vi "UHR-Fleezers Control (host) -TL - oscillation.vi"(0 "Tab Control":T5(tab)) -> ()   [LabVIEW 2013] (continued)
            n248 = VISA Write(VISA resource name=w463, write buffer=w464) -> ()  [unwired: 1 in, 3 out]
          }
          frame #4 {
            n249 = Wait (ms)(milliseconds to wait=u32 200) -> ()  [unwired: 1 out]
          }
          frame #5 {
            # "Change the trajectory mode to Jog"
            n250 = local read "ESP Port"() -> (w468:refnum<visa-resource-name>)
            n251 = Concatenate Strings("1TJ3;\n2TJ3;\n3TJ3" ("Substring"), "\r") -> (w471:string)
            n252 = VISA Write(VISA resource name=w468, write buffer=w471) -> ()  [unwired: 1 in, 3 out]
          }
        }
      }
      event "Capture": Value Change {
        n253 = event-data() -> ()  [unwired: 1 in, 5 out]
        n254 = local read "Capture Locations"() -> (w472:i32)
        n255 = local read "Z Pos Pos"() -> (w473:string)
        n256 = local read "X Pos"() -> (w475:string)
        n257 = local read "Y Pos"() -> (w474:string)
        n258 = case shown="1" w472 {
          selector: w472 -> [w479 w486 w493 w500]
          tunnel: w475 -> [w482 w489 w496 w503]
          tunnel: w474 -> [w481 w488 w495 w502]
          tunnel: w473 -> [w480 w487 w494 w501]
          frame 0, Default {
            # "Capture Top Dispensor Location"
            n259 = local read "Location Matrix"() -> (w478:string[][])
            n260 = Build Array(w482, w481, w480) -> (w477:string[])
            n261 = Replace Array Subset(array=w478, new element=w477, index (row)=w479) -> (w476:string[][])  [unwired: 1 in]
            n262 = local write "Location Matrix"(w476) -> ()
          }
          frame 1 {
            # "Capture Bottom Dispensor Location"
            n263 = local read "Location Matrix"() -> (w485:string[][])
            n264 = Build Array(w489, w488, w487) -> (w484:string[])
            n265 = Replace Array Subset(array=w485, new element=w484, index (row)=w486) -> (w483:string[][])  [unwired: 1 in]
            n266 = local write "Location Matrix"(w483) -> ()
          }
          frame 2 {
            # "Capture Experimental Region Location"
            n267 = local read "Location Matrix"() -> (w492:string[][])
            n268 = Build Array(w496, w495, w494) -> (w491:string[])
            n269 = Replace Array Subset(array=w492, new element=w491, index (row)=w493) -> (w490:string[][])  [unwired: 1 in]
            n270 = local write "Location Matrix"(w490) -> ()
          }
          frame 3 {
            # "Capture Other Location"
            n271 = local read "Location Matrix"() -> (w499:string[][])
            n272 = Build Array(w503, w502, w501) -> (w498:string[])
            n273 = Replace Array Subset(array=w499, new element=w498, index (row)=w500) -> (w497:string[][])  [unwired: 1 in]
            n274 = local write "Location Matrix"(w497) -> ()
          }
        }
      }
      event "Save": Value Change {
        # "reshape Location Matrix to 1-D array to write"
        n275 = event-data() -> ()  [unwired: 1 in, 5 out]
        n276 = local read "Location Matrix"() -> (w507:string[][])
        n277 = local read "Location path"() -> (w504:path)
        n278 = Reshape Array(w507, 12) -> (w505:string[])
        n279 = Write to Text File(file (use dialog)=w504, text=w505) -> ()  [unwired: 2 in, 3 out]
      }
      event "Activate Joystick": Value Change {
        # "Change the trajectory mode to Jog"
        n280 = event-data() -> ()  [unwired: 1 in, 5 out]
        n281 = disable-structure shown="Disabled" {
          frame Disabled {
            n282 = case shown="True" "Activate Joystick" {
              frame False {
              }
              frame True {
                # "Change the trajectory mode to Jog"
                n283 = local read "ESP Port"() -> (w516:refnum<visa-resource-name>)
                n284 = Concatenate Strings("1TJ3;\n2TJ3;\n3TJ3" ("Substring"), "\r") -> (w513:string)
                n285 = VISA Write(VISA resource name=w516, write buffer=w513) -> ()  [unwired: 1 in, 3 out]
              }
            }
          }
          frame Enabled {
          }
        }
        n286 = local read "ESP Port"() -> (w508:refnum<visa-resource-name>)
        n287 = Concatenate Strings("1TJ3;\n2TJ3;\n3TJ3" ("Substring"), "\r") -> (w511:string)
        n288 = VISA Write(VISA resource name=w508, write buffer=w511) -> ()  [unwired: 1 in, 3 out]
      }
    }
  }
  n289 = disable-structure shown="Disabled" {
    disable-tunnel: w2 -> [w545 _]
    frame Disabled {
      w540 = T17 0 items=["Grayscale (U8)", "Grayscale (I16)", "Grayscale (SGL)", "Complex (CSG)", "RGB (U32)", "HSL (U32)", "RGB (U64)", "Grayscale (U16)"] ("Image Type")
      n290 = call <vilib>:"IMAQ Init.vi"("Interface Name"="img0") -> ("error out"=w542:errorcluster, "IMAQ Session Out"=w544:refnum<k11>)  [unwired: 9 in]
      n291 = call <vilib>:"IMAQ Grab Setup.vi"("error in (no error)"=w542, "IMAQ Session In"=w544) -> ("error out"=w538:errorcluster, "IMAQ Session Out"=w539:refnum<k11>)  [unwired: 8 in]
      n292 = call "IMAQ Create"("Image Name"="untitled", "Image Type"=w540) -> ("New Image"=w537:T3)  [unwired: 3 in, 1 out]
      n293 = call <vilib>:"Application Directory.vi"() -> ("Application Directory"=w524:path)
      n294 = Build Path(base path=w524, name or relative path="_trap_screen_positions") -> (appended path=w532:path)
      n295 = Open/Create/Replace File(file path (use dialog)=w532, operation (0:open)=T23."open or create", access (0:read/write)=enum16{"read/write", "read-only", "write-only"}."read/write") -> (refnum out=w534:refnum<file>)  [unwired: 3 in, 2 out]
      n296 = local read "Trap Sets"() -> (w526:u32)
      n297 = for "Load trap positions on video screen from file." {
        N: w526 -> [_]
        tunnel: [w552] -> w527
        tunnel: w534 -> [w551]
        tunnel: [w548] -> w523 mode=indexing
        w550 = 4
        n298 = for {
          N: w550 -> [_]
          tunnel: [w556] -> w552
          tunnel: w551 -> [w555]
          tunnel: w550 -> [w554]
          tunnel: [w553] -> w549 mode=indexing
          n299 = Read from Binary File(5:w554, 11:w555) -> (2:w553:i32, 3:w556:refnum<file>)  [unwired: 4 in, 2 out]
        }
        n300 = Array To Cluster(array=w549) -> (cluster=w548:T27)
      }
      n301 = node-c288() -> (w547:T24)  [unwired: 4 in]
      n302 = timed-loop "acquire video and stage position" {
        timing: w547 -> [_]
        timing-out: [_] -> w546
        tunnel: w539 -> [w575]
        tunnel: w538 -> [w574]
        tunnel: w537 -> [w573]
        tunnel: [w572] -> w519
        tunnel: [w569] -> w520
        tunnel: [w570] -> w518
        tunnel: w545 -> [_]
        shift-right: [w566] -> w536
        shift-left: w523 -> [w567]
        tunnel: w526 -> [w564]
        stop <- w571 stop-if-true
        n303 = node-c288() -> ()  [unwired: 1 in, 1 out]
        n304 = event shown="[0] Timeout" {
          selector: _ -> [_ _ _ _]
          dyn-events: _ -> [_ _ _ _]
          timeout: 10 -> [_ _ _ _]
          tunnel: w575 -> [w586 w601 w610 w629]
          tunnel: w574 -> [w585 w603 w608 w631]
          tunnel: w573 -> [w584 w602 w609 w630]
          tunnel: [w583 w601 w610 w629] -> w572
          tunnel: [w576 w605 FALSE FALSE] -> w571
          tunnel: [w580 w603 w608 w631] -> w570
          tunnel: [w579 w602 w609 w630] -> w569
          tunnel: "radius" -> [_ _ w615 _]
          tunnel: w567 -> [w577 w604 w613 _]
          tunnel: [w577 w604 w614 cluster{i32, i32, i32, i32}[] []] -> w566
          tunnel: w564 -> [_ _ w606 _]
          event Timeout {
            n305 = event-data() -> ()  [unwired: 1 in, 2 out]
            n306 = call <vilib>:"IMAQ Grab Acquire.vi"("error in (no error)"=w585, "Image In"=w584, "IMAQ Session In"=w586) -> ("error out"=w581:errorcluster, "Image Out"=w582:T3, "IMAQ Session Out"=w583:refnum<k11>)  [unwired: 5 in, 1 out]
            n307 = case shown="True" "trap\nmarkers?" {
              tunnel: w577 -> [_ w594]
              tunnel: w582 -> [w588 w593]
              tunnel: w581 -> [w587 w592]
              tunnel: [w587 w591] -> w580
              tunnel: [w588 w589] -> w579
              frame False {
              }
              frame True {
                n308 = for {
                  tunnel: w594 -> [w600] mode=indexing
                  shift-right: [w598] -> w589
                  shift-left: w593 -> [w599]
                  tunnel: w592 -> [w597]
                  tunnel: [w596] -> w591
                  tunnel: u32 16711680 ("Color") -> [w595]
                  n309 = call "IMAQ Overlay Oval"("Color"=w595, "error in (no error)"=w597, "Bounding Rectangle"=w600, "Image"=w599) -> ("error out"=w596:errorcluster, "Image Out"=w598:T3)  [unwired: 6 in]
                }
              }
            }
            "Primary Video Display" <- w579
            n310 = Unbundle By Name(w581) -> ("status"=w576:bool)
          }
          event "Stop All": Value Change {
            n311 = event-data() -> ()  [unwired: 1 in, 5 out]
            n312 = local read "Stop All"() -> (w605:bool)
          }
          event "Primary Video Display": Mouse Down {
            n313 = event-data() -> ()  [unwired: 1 in, 7 out]
            n314 = Array Size(array=w613) -> (size(s)=w612:i32)
            n315 = Less?(x=w612, y=w606) -> (x < y?=w611:bool)
            n316 = case shown="True" w611 {
              tunnel: w615 -> [_ w625]
              tunnel: w613 -> [w616 w619]
              tunnel: [w616 w618] -> w614
              frame False {
              }
              frame True {
                n317 = property on="Primary Video Display" class="ImageControl"() -> ("Last Mouse Position"=w617:cluster{"X":i32, "Y":i32})  [unwired: 2 in, 2 out]
                n318 = Unbundle By Name(w617) -> ("X"=w627:i32, "Y"=w626:i32)
                n319 = Add(x=w626, y=w625) -> (x+y=w623:i32)
                n320 = Subtract(x=w626, y=w625) -> (x-y=w621:i32)
                n321 = Add(x=w627, y=w625) -> (x+y=w622:i32)
                n322 = Subtract(x=w627, y=w625) -> (x-y=w624:i32)
                n323 = Bundle(w624, w623, w622, w621) -> (w620:cluster{i32, i32, i32, i32})  [unwired: 1 in]
                n324 = Build Array (concatenate)(w619, w620) -> (w618:T28)
              }
            }
          }
          event "clear markers": Value Change {
            n325 = event-data() -> ()  [unwired: 1 in, 5 out]
          }
        }
        n326 = node-c288() -> ()  [unwired: 1 in, 1 out]
      }
      n327 = node-c288(w546) -> ()  [unwired: 1 out]
      n328 = Set File Position(offset (in bytes) (0)=i64 0, refnum=w527, from (0:start)=enum16{"start", "end", "current"}."start") -> (refnum out=w528:refnum<file>)  [unwired: 1 in, 1 out]
      n329 = for "Write trap positions to file so they can be remembered\nwhen program is removed from memory" {
        tunnel: w536 -> [w560] mode=indexing
        tunnel: [w558] -> w535
        tunnel: w528 -> [w557]
        n330 = Cluster To Array(cluster=w560) -> (array=w559:i32[])
        n331 = for {
          tunnel: w559 -> [w563] mode=indexing
          tunnel: [w562] -> w558
          tunnel: w557 -> [w561]
          n332 = Write to Binary File(file (use dialog)=w561, data=w563) -> (refnum out=w562:refnum<file>)  [unwired: 4 in, 2 out]
        }
      }
      n333 = Close File(refnum=w535) -> ()  [unwired: 1 in, 2 out]
      n334 = call "IMAQ Dispose"("Image"=w520, "error in (no error)"=w518) -> ("error out"=w517:errorcluster)  [unwired: 4 in]
      n335 = call <vilib>:"IMAQ Stop.vi"("error in (no error)"=w517, "IMAQ Session In"=w519) -> ("error out"=w521:errorcluster, "IMAQ Session Out"=w522:refnum<k11>)  [unwired: 8 in]
      n336 = call <vilib>:"IMAQ Close.vi"("error in (no error)"=w521, "IMAQ Session In"=w522) -> ()  [unwired: 9 in, 1 out]
    }
    frame Enabled {
    }
  }
  n337 = disable-structure shown="Enabled" {
    disable-tunnel: [w638 _] -> w39
    disable-tunnel: w2 -> [w637 _]
    frame Enabled {
      n338 = node-c288() -> (w640:T24)  [unwired: 4 out]
      n339 = timed-loop "Rough control of MCL mirror stage (debugging)" {
        tunnel: w637 -> [w643]
        tunnel: [w642] -> w638
        timing: w640 -> [_]
        timing-out: [_] -> w639
        stop <- w642 stop-if-true
        n340 = node-c288() -> ()  [unwired: 2 out]
        n341 = case shown="1" "MCL Mode" {
          tunnel: w643 -> [_ w646 w693]
          frame 0, Default {
            # "manual positioning"
          }
          frame 1 {
            # "sinusoidal wave"
            n342 = node-c288() -> (w648:T24)  [unwired: 4 out]
            n343 = timed-loop "Oscillate MCL mirror" {
              timing: w648 -> [_]
              timing-out: [_] -> w647
              tunnel: w646 -> [w687]
              i -> [w686]
              stop <- w649 stop-if-true
              n344 = node-c288() -> (w685:i64)  [unwired: 1 out]
              n345 = Multiply(x="AO1", y=32767.0) -> (x*y=w681:dbl)
              n346 = Multiply(x="AO2", y=32767.0) -> (x*y=w676:dbl)
              n347 = Divide(x=w681, y=10.0) -> (x/y=w682:dbl)
              n348 = Divide(x=w676, y=10.0) -> (x/y=w677:dbl)
              n349 = To Word Integer(number=w682) -> (16bit integer=w674:i16)
              n350 = To Word Integer(number=w677) -> (16bit integer=w673:i16)
              n351 = Divide(x=w685, y=i64 1000) -> (x/y=w656:dbl)
              n352 = Multiply(x=w656, y=w686) -> (x*y=w667:dbl)
              n353 = Multiply(x="Osc. freq. (Hz) 2", y=6.283185307179586) -> (x*y=w668:dbl)
              n354 = Multiply(x=w668, y=w667) -> (x*y=w666:dbl)
              n355 = Sine(x=w666) -> (sin(x)=w665:dbl)
              n356 = Multiply(x=w665, y="Osc. amp. (V)") -> (x*y=w663:dbl)
              n357 = Add(x=w663, y="Osc. center (V)") -> (x+y=w661:dbl)
              n358 = Divide(x=w661, y=10.0) -> (x/y=w659:dbl)
              n359 = Multiply(x=w659, y=32767.0) -> (x*y=w654:dbl)
              n360 = Select(t=w654, s="Scan axis", f=w674) -> (s? t:f=w672:dbl)
              n361 = Select(t=w673, s="Scan axis", f=w654) -> (s? t:f=w671:dbl)
              n362 = local read "MCL Mode"() -> (w653:u16)
              n363 = Not Equal?(x=w653, y=u16 1) -> (x != y?=w650:bool)
              n364 = local read "Stop All"() -> (w651:bool)
              n365 = xnode "Read/Write Control"("FPGA VI Reference In"=w687, "AO1"=w672, "AO2"=w671) -> ()  [unwired: 1 in, 2 out]
              n366 = Compound Arithmetic op=OR(w651, w650) -> (w649:bool)
              n367 = node-c288() -> ()  [unwired: 2 out]
            }
            n368 = node-c288(w647) -> ()  [unwired: 1 out]
          }
          frame 2 {
            # "linear scan"
            n369 = case shown="True" "Start Scan" {
              tunnel: w693 -> [_ w705]
              frame False {
              }
              frame True {
                n370 = Subtract(x="End (V)", y="Begin (V)") -> (x-y=w701:dbl)
                n371 = Decrement(x="N Points") -> (x-1=w700:dbl)
                n372 = Divide(x=w701, y=w700) -> (x/y=w698:dbl)
                n373 = for {
                  N: "N Points" -> [_]
                  tunnel: "Begin (V)" -> [w718]
                  tunnel: w705 -> [w710]
                  tunnel: [w709] -> w704 mode=indexing
                  tunnel: w698 -> [w708]
                  tunnel: [w706] -> w697 mode=indexing
                  i -> [w717]
                  n374 = Multiply(x=w708, y=w717) -> (x*y=w716:dbl)
                  n375 = Add(x=w718, y=w716) -> (x+y=w713:dbl)
                  n376 = local read "Scan axis"() -> (w707:bool)
                  n377 = local read "AO1"() -> (w715:dbl)
                  n378 = local read "AO2"() -> (w714:dbl)
                  n379 = Select(t=w713, s=w707, f=w715) -> (s? t:f=w712:dbl)
                  n380 = Select(t=w714, s=w707, f=w713) -> (s? t:f=w711:dbl)
                  n381 = flat-sequence {
                    tunnel: w712 -> [w722]
                    tunnel: w711 -> [w721]
                    tunnel: w710 -> [w719]
                    tunnel: [w732] -> w709
                    tunnel: [w731] -> w706
                    frame #0 {
                      w725 = 10.0 ("y")
                      w720 = 32767.0 ("y")
                      n382 = Multiply(x=w722, y=w720) -> (x*y=w728:dbl)
                      n383 = Multiply(x=w721, y=w720) -> (x*y=w726:dbl)
                      n384 = Divide(x=w728, y=w725) -> (x/y=w729:dbl)
                      n385 = Divide(x=w726, y=w725) -> (x/y=w727:dbl)
                      n386 = To Word Integer(number=w729) -> (16bit integer=w723:i16)
                      n387 = To Word Integer(number=w727) -> (16bit integer=w724:i16)
                      n388 = xnode "Read/Write Control"("FPGA VI Reference In"=w719, "AO1"=w723, "AO2"=w724) -> ()  [unwired: 1 in, 2 out]
                    }
                    frame #1 {
                      n389 = Wait (ms)(milliseconds to wait="DAQ Delay (ms)") -> ()  [unwired: 1 out]
                    }
                    frame #2 {
                      n390 = local read "Slow mean"() -> (w732:dbl)
                      n391 = local read "Sigma"() -> (w731:dbl)
                    }
                  }
                }
                n392 = Bundle("Begin (V)"="Begin (V)", w698, w704) -> (→"MCL Scan":cluster{"Begin (V)":dbl, dbl, dbl[]})  [unwired: 1 out]
                n393 = Bundle("Begin (V)"="Begin (V)", w698, w697) -> (→"MCL Scan 2":cluster{"Begin (V)":dbl, dbl, dbl[]})  [unwired: 1 out]
              }
            }
          }
        }
        n394 = local read "Stop All"() -> (w642:bool)
        n395 = node-c288() -> ()  [unwired: 2 out]
      }
      n396 = node-c288(w639) -> ()  [unwired: 1 out]
    }
    frame Disabled {
    }
  }
  n397 = node-c288(i64 100 ("Period")) -> (w72:T24)  [unwired: 3 in]
  n398 = timed-loop "Run Scripts, including: stage motion" {
    timing: w72 -> [_]
    timing-out: [_] -> w71
    tunnel: w2 -> [w735]
    stop <- w737 stop-if-true
    n399 = node-c288() -> ()  [unwired: 1 in, 1 out]
    n400 = event shown="[2] \"Cal/Data Acq. Spot\": Value Change" {
      selector: _ -> [_ _ _ _ _ _ _ _ _ _ _ _]
      dyn-events: _ -> [_ _ _ _ _ _ _ _ _ _ _ _]
      timeout: 50 -> [_ _ _ _ _ _ _ _ _ _ _ _]
      tunnel: ["Move Cap. 1 (DNA Top)" _ "Cal/Data Acq. Spot" "Dump Beads" "Dip for Protein" _ "Got ADig bead" "Got DNA bead" "Take Stepping Data" _ "Take Detection Laser\nImage" _] -> _
      tunnel: [_ _ _ _ _ _ _ _ _ _ _ w947] -> w737
      tunnel: w735 -> [_ _ _ _ _ _ _ _ _ _ _ _]
      event "Move Cap. 1 (DNA Top)": Value Change {
        n401 = event-data() -> ()  [unwired: 1 in, 5 out]
        n402 = local write "Move Cap. 1 (DNA Top)"(FALSE ("Move Cap. 1 (DNA Right)")) -> ()
        n403 = flat-sequence {
          tunnel: "Cap 1 Samp Flow ON" -> [w743]
          frame #0 {
            n404 = local write "Stage Moving"(FALSE ("Stage Moving")) -> ()
            n405 = case "stop flow" shown="True" w743 {
              frame False {
              }
              frame True {
                n406 = call "hamilton_controller.vi"("Open?"=FALSE, "valve"=enum16{"A", "B", "C", "D", "ALL"}."C", "action"=T20."MOVE VALVE") -> ()  [unwired: 8 in, 1 out]
              }
            }
            n407 = case shown="True" TRUE {
              tunnel: "Cap 1 T ON" -> [w752 w753]
              frame False {
                n408 = property on="Trap 1 (ON/OFF)" class="Bool (strict)"("Val(Sgnl)"=w752) -> ()  [unwired: 2 in, 2 out]
              }
              frame True {
                n409 = property on="Trap 2 (ON/OFF)" class="Bool (strict)"("Val(Sgnl)"=w753) -> ()  [unwired: 2 in, 2 out]
              }
            }
            n410 = call <vilib>:"Beep.vi"() -> ()  [unwired: 3 in, 9 out]
            n411 = case shown="True" "Cap 1 Flow ON" {
              frame False {
              }
              frame True {
                n412 = property on="Inject Top:" class="Bool (strict)"("Val(Sgnl)"=TRUE ("Value (Signaling)")) -> ()  [unwired: 2 in, 2 out]
              }
            }
          }
        }
      }
      event Timeout {
        n413 = event-data() -> ()  [unwired: 1 in, 2 out]
      }
      event "Cal/Data Acq. Spot": Value Change {
        # "wait for calibration file\nto be written"
        # "signal save cal true\nthis tells the data \nacquisition loop to\nstart sending the data\nto a calibration file"
        # "separate traps to\nthe desired trap delta"
        # "move stage to data acquisition spot"
        # "CHANGE FISH FOR TETHER BACK\nTO TRUE VALUE HERE."
        n414 = event-data() -> ()  [unwired: 1 in, 5 out]
        n415 = local write "Cal/Data Acq. Spot"(FALSE ("Cal/Data Acq. Spot")) -> ()
        n416 = flat-sequence {
          tunnel: ["Cal @ (MHz)"] -> w754
          tunnel: w754 -> [w765]
          tunnel: w754 -> [w786]
          frame #0 {
            n417 = property on="Trap Delta (MHz)" class="DigNum (strict)"("Val(Sgnl)"="Cal @ (MHz)") -> ()  [unwired: 2 in, 2 out]
            n418 = call <vilib>:"Beep.vi"() -> ()  [unwired: 3 in, 9 out]
          }
          frame #1 {
            n419 = property on="Oscillate Traps\n(during calibration)" class="Bool (strict)"("Val(Sgnl)"=TRUE ("Oscillate Set 2")) -> ()  [unwired: 2 in, 2 out]
          }
          frame #2 {
            n420 = Wait (ms)(milliseconds to wait=u32 100) -> ()  [unwired: 1 out]
          }
          frame #3 {
            n421 = property on="Save Calibration" class="Bool (strict)"("Val(Sgnl)"=TRUE ("Value (Signaling)")) -> ()  [unwired: 2 in, 2 out]
          }
          frame #4 {
            n422 = Wait (ms)(milliseconds to wait=u32 4000) -> ()  [unwired: 1 out]
          }
          frame #5 {
            n423 = while {
              stop <- w762 stop-if-true
              n424 = local read "Saving..."() -> (w763:bool)
              n425 = Wait (ms)(milliseconds to wait=u32 100) -> ()  [unwired: 1 out]
              n426 = Not(x=w763) -> (.not. x?=w762:bool)
            }
          }
          frame #6 {
            n427 = case shown="True" "W/ Offset 1" {
              tunnel: w765 -> [_ w767]
              frame False {
              }
              frame True {
                n428 = stacked-sequence {
                  tunnel: w767 -> [_ _ _ _ _ _ _ w784]
                  frame #0 {
                    n429 = Replace Array Subset(array=u32[] [0] ("Index Values"), new element="Offset 1 Set", index=0) -> (w768:u32[])
                    n430 = property on="Saved AOD Raster Scan Parameter Sets" class="Arr (strict)"("Index Values"=w768) -> ()  [unwired: 2 in, 2 out]
                    n431 = property on="Trap Delta (MHz)" class="DigNum (strict)"("Val(Sgnl)"="Offset 1 Start (MHz)") -> ()  [unwired: 2 in, 2 out]
                  }
                  frame #1 {
                    n432 = Wait (ms)(milliseconds to wait=u32 200) -> ()  [unwired: 1 out]
                  }
                  frame #2 {
                    n433 = property on="Load parameters" class="Bool (strict)"("Val(Sgnl)"=TRUE ("Value (Signaling)")) -> ()  [unwired: 2 in, 2 out]
                  }
                  frame #3 {
                    n434 = Wait (ms)(milliseconds to wait=u32 200) -> ()  [unwired: 1 out]
                  }
                  frame #4 {
                    n435 = property on="Trap Raster Scan" class="Bool (strict)"("Val(Sgnl)"=TRUE ("Value (Signaling)")) -> ()  [unwired: 2 in, 2 out]
                  }
                  frame #5 {
                    n436 = Wait (ms)(milliseconds to wait=u32 2000) -> ()  [unwired: 1 out]
                  }
                  frame #6 {
                    n437 = while {
                      stop <- w781 stop-if-true
                      n438 = local read "Raster Scanning..."() -> (w783:bool)
                      n439 = local read "Saving..."() -> (w779:bool)
                      n440 = Wait (ms)(milliseconds to wait=u32 100) -> ()  [unwired: 1 out]
                      n441 = Not(x=w779) -> (.not. x?=w778:bool)
                      n442 = Not(x=w783) -> (.not. x?=w780:bool)
                      n443 = And(x=w780, y=w778) -> (x .and. y?=w781:bool)
                    }
                  }
                  frame #7 {
                    n444 = property on="Trap Delta (MHz)" class="DigNum (strict)"("Val(Sgnl)"=w784) -> ()  [unwired: 2 in, 2 out]
                  }
                }
              }
            }
          }
          frame #7 {
            n445 = local read "Save ave N"() -> (w785:dbl)
            n446 = case shown="True" "W/ Offset 2" {
              tunnel: w786 -> [_ w792]
              tunnel: w785 -> [_ w791]
              frame False {
                n447 = Multiply(x="Cal read wait (s)", y=u32 1000 ("milliseconds to wait")) -> (x*y=w789:u32)
                n448 = Wait (ms)(milliseconds to wait=w789) -> ()  [unwired: 1 out]
              }
              frame True {
                n449 = stacked-sequence {
                  tunnel: w792 -> [_ _ _ _ _ _ _ _ _ w813 _ _]
                  tunnel: w791 -> [_ _ _ _ _ _ _ _ _ w811 _ _]
                  frame #0 {
                    n450 = property on="Save ave N" class="DigNum (strict)"("Val(Sgnl)"=1.0 ("Value (Signaling)")) -> ()  [unwired: 2 in, 2 out]
                  }
                  frame #1 {
                    n451 = Wait (ms)(milliseconds to wait=u32 500) -> ()  [unwired: 1 out]
                  }
                  frame #2 {
                    n452 = property on="Trap Delta (MHz)" class="DigNum (strict)"("Val(Sgnl)"="Offset 2 Start (MHz)") -> ()  [unwired: 2 in, 2 out]
                    n453 = Replace Array Subset(array=u32[] [0] ("Index Values"), new element="Offset 2 Set", index=0) -> (w797:u32[])
                    n454 = property on="Saved AOD Raster Scan Parameter Sets" class="Arr (strict)"("Index Values"=w797) -> ()  [unwired: 2 in, 2 out]
                  }
                  frame #3 {
                    n455 = Wait (ms)(milliseconds to wait=u32 500) -> ()  [unwired: 1 out]
                  }
                  frame #4 {
                    n456 = property on="Load parameters" class="Bool (strict)"("Val(Sgnl)"=TRUE ("Value (Signaling)")) -> ()  [unwired: 2 in, 2 out]
                  }
                  frame #5 {
                    n457 = Wait (ms)(milliseconds to wait=u32 500) -> ()  [unwired: 1 out]
                  }
                  frame #6 {
                    n458 = property on="Trap Raster Scan" class="Bool (strict)"("Val(Sgnl)"=TRUE ("Value (Signaling)")) -> ()  [unwired: 2 in, 2 out]
                  }
                  frame #7 {
                    n459 = Wait (ms)(milliseconds to wait=u32 2000) -> ()  [unwired: 1 out]
                  }
                  frame #8 {
                    n460 = while {
                      stop <- w806 stop-if-true
                      n461 = local read "Raster Scanning..."() -> (w809:bool)
                      n462 = local read "Saving..."() -> (w807:bool)
                      n463 = Wait (ms)(milliseconds to wait=u32 100) -> ()  [unwired: 1 out]
                      n464 = Not(x=w807) -> (.not. x?=w805:bool)
                      n465 = Not(x=w809) -> (.not. x?=w808:bool)
                      n466 = And(x=w808, y=w805) -> (x .and. y?=w806:bool)
                    }
                  }
                  frame #9 {
                    n467 = property on="Trap Delta (MHz)" class="DigNum (strict)"("Val(Sgnl)"=w813) -> ()  [unwired: 2 in, 2 out]
                    n468 = property on="Saved AOD Raster Scan Parameter Sets" class="Arr (strict)"("Index Values"=u32[] [0]) -> ()  [unwired: 2 in, 2 out]
                    n469 = property on="Save ave N" class="DigNum (strict)"("Val(Sgnl)"=w811) -> ()  [unwired: 2 in, 2 out]
                  }
                  frame #10 {
                    n470 = Wait (ms)(milliseconds to wait=u32 500) -> ()  [unwired: 1 out]
                  }
                  frame #11 {
                    n471 = property on="Load parameters" class="Bool (strict)"("Val(Sgnl)"=TRUE ("Value (Signaling)")) -> ()  [unwired: 2 in, 2 out]
                  }
                }
              }
            }
          }
          frame #8 {
            n472 = property on="Read Cal" class="Bool (strict)"("Val(Sgnl)"=TRUE ("Value (Signaling)")) -> ()  [unwired: 2 in, 2 out]
          }
          frame #9 {
            n473 = Wait (ms)(milliseconds to wait=u32 500) -> ()  [unwired: 1 out]
          }
          frame #10 {
            n474 = property on="Fish for Tether" class="Bool (strict)"("Val(Sgnl)"=FALSE ("Value (Signaling)")) -> ()  [unwired: 2 in, 2 out]
          }
          frame #11 {
            n475 = property on="Oscillate Traps\n(during calibration)" class="Bool (strict)"("Val(Sgnl)"=FALSE ("Oscillate Set 2")) -> ()  [unwired: 2 in, 2 out]
          }
        }
      }
      event "Dump Beads": Value Change {
        # "SCRIPT TO REMOVE BOTH BEADS FROM THE TRAPS. TURNS ON LIGHT WHICH INDICATES THAT STAGE IS MOVING. THEN STOPS SAVING DATA. \nSETS Sample Channel Flow TO TRUE. STOPS INTERLACING GREEN FLUORESCENCE. TURNS OFF Tether INDICATOR BECAUSE WE ARE THROWING IT\nAWAY. SHUTS OFF TRAP POSITION FEEDBACK."
        n476 = event-data() -> ()  [unwired: 1 in, 5 out]
        n477 = flat-sequence {
          frame #0 {
            w821 = FALSE ("Fl. Triggered...")
            w822 = TRUE ("Stage Moving")
            n478 = local read "Saving..."() -> (w823:bool)
            n479 = local write "Fl. Triggered..."(w821) -> ()
            n480 = local write "Stage Moving"(w822) -> ()
            n481 = local write "Tether"(w821) -> ()
            n482 = property on="Green Laser ON/Interlacing" class="Bool (strict)"("Val(Sgnl)"=w821) -> ()  [unwired: 2 in, 2 out]
            n483 = property on="Trap Pos. FB ON" class="Bool (strict)"("Val(Sgnl)"=w821) -> ()  [unwired: 2 in, 2 out]
            n484 = property on="Main:" class="Bool (strict)"("Val(Sgnl)"=w822) -> ()  [unwired: 2 in, 2 out]
            n485 = local write "Stop Saving"(w823) -> ()
          }
          frame #1 {
            w824 = FALSE ("Value (Signaling)")
            # "TURNS TRAPS OFF SO THAT\nBEADS REMAIN AT DUMP \nBEADS POSITION"
            n486 = property on="Trap 1 (ON/OFF)" class="Bool (strict)"("Val(Sgnl)"=w824) -> ()  [unwired: 2 in, 2 out]
            n487 = property on="Trap 2 (ON/OFF)" class="Bool (strict)"("Val(Sgnl)"=w824) -> ()  [unwired: 2 in, 2 out]
            n488 = call <vilib>:"Beep.vi"() -> ()  [unwired: 3 in, 9 out]
          }
          frame #2 {
            n489 = property on="Goto Bottom (F7)" class="Bool (strict)"("Val(Sgnl)"=TRUE ("Value (Signaling)")) -> ()  [unwired: 2 in, 2 out]
          }
          frame #3 {
            n490 = Wait (ms)(milliseconds to wait=u32 8000) -> ()  [unwired: 1 out]
          }
          frame #4 {
            n491 = property on="Trap Delta (MHz)" class="DigNum (strict)"("Val(Sgnl)"=20.0 ("Value (Signaling)")) -> ()  [unwired: 2 in, 2 out]
          }
          frame #5 {
            n492 = property on="Trap 2 (ON/OFF)" class="Bool (strict)"("Val(Sgnl)"=TRUE ("Value (Signaling)")) -> ()  [unwired: 2 in, 2 out]
          }
          frame #6 {
            n493 = property on="Main:" class="Bool (strict)"("Val(Sgnl)"=FALSE ("Value (Signaling)")) -> ()  [unwired: 2 in, 2 out]
          }
        }
      }
      event "Dip for Protein": Value Change {
        n494 = event-data() -> ()  [unwired: 1 in, 5 out]
        n495 = flat-sequence {
          frame #0 {
            n496 = case shown="True" "Move Trap Before?" {
              frame False {
              }
              frame True {
                n497 = property on="Trap Delta (MHz)" class="DigNum (strict)"("Val(Sgnl)"="Dip Trap Delta 1 (MHz)") -> ()  [unwired: 2 in, 2 out]
              }
            }
          }
          frame #1 {
            n498 = Multiply(x="Duration (s)", y=1000.0) -> (x*y=w833:dbl)
            n499 = Wait (ms)(milliseconds to wait=w833) -> ()  [unwired: 1 out]
          }
          frame #2 {
            n500 = case shown="True" "Move Trap After?" {
              frame False {
              }
              frame True {
                n501 = property on="Trap Delta (MHz)" class="DigNum (strict)"("Val(Sgnl)"="Dip Trap Delta 2 (MHz)") -> ()  [unwired: 2 in, 2 out]
              }
            }
          }
          frame #3 {
            n502 = case shown="True" "Green ON After?" {
              frame False {
              }
              frame True {
                n503 = property on="Green Laser ON/Interlacing" class="Bool (strict)"("Val(Sgnl)"=TRUE ("Value (Signaling)")) -> ()  [unwired: 2 in, 2 out]
              }
            }
          }
          frame #4 {
            n504 = Wait (ms)(milliseconds to wait=u32 500) -> ()  [unwired: 1 out]
          }
          frame #5 {
            n505 = case shown="True" "Save Data After?" {
              frame False {
              }
              frame True {
                n506 = property on="Start Saving" class="Bool (strict)"("Val(Sgnl)"=TRUE ("Value (Signaling)")) -> ()  [unwired: 2 in, 2 out]
              }
            }
          }
        }
      }
      event "Profile": Value Change {
        n507 = event-data() -> ()  [unwired: 1 in, 5 out]
        n508 = flat-sequence {
          frame #0 {
            w843 = 0.0 ("element")
            n509 = Build Array(w843, "Y change (mm)", w843) -> ()  [unwired: 1 out]
          }
          frame #1 {
            # "stop saving"
            n510 = local write "Stop Saving"(TRUE ("Stop Saving")) -> ()
            n511 = local write "Stage Moving"(FALSE ("Stage Moving")) -> ()
          }
        }
      }
      event "Got ADig bead": Value Change {
        n512 = event-data() -> ()  [unwired: 1 in, 5 out]
        n513 = property on="Move Cap. 1 (DNA Top)" class="Bool (strict)"("Val(Sgnl)"=TRUE ("Value (Signaling)")) -> ()  [unwired: 2 in, 2 out]
        n514 = property on="Inject Bottom:" class="Bool (strict)"("Val(Sgnl)"=FALSE ("Value (Signaling)")) -> ()  [unwired: 2 in, 2 out]
      }
      event "Got DNA bead": Value Change {
        n515 = event-data() -> ()  [unwired: 1 in, 5 out]
        n516 = property on="Cal/Data Acq. Spot" class="Bool (strict)"("Val(Sgnl)"=TRUE ("Value (Signaling)")) -> ()  [unwired: 2 in, 2 out]
        n517 = property on="Inject Top:" class="Bool (strict)"("Val(Sgnl)"=FALSE ("Value (Signaling)")) -> ()  [unwired: 2 in, 2 out]
      }
      event "Take Stepping Data": Value Change {
        n518 = event-data() -> ()  [unwired: 1 in, 5 out]
        n519 = local read "Save ave N"() -> (w861:dbl)
        n520 = flat-sequence {
          tunnel: w861 -> [w863]
          tunnel: [w863] -> w856
          tunnel: [w865] -> w857
          tunnel: w856 -> [w865]
          tunnel: [w867] -> w858
          tunnel: w857 -> [w867]
          tunnel: [w870] -> w859
          tunnel: w858 -> [w870]
          tunnel: [w872] -> w860
          tunnel: w859 -> [w872]
          tunnel: [w874] -> w854
          tunnel: w860 -> [w874]
          tunnel: w854 -> [w877]
          tunnel: [w877] -> w853
          tunnel: w853 -> [w878]
          tunnel: [w878] -> w855
          tunnel: w855 -> [w884]
          frame #0 {
            n521 = property on="Save ave N" class="DigNum (strict)"("Val(Sgnl)"="Save ave factor") -> ()  [unwired: 2 in, 2 out]
          }
          frame #1 {
            n522 = Wait (ms)(milliseconds to wait=u32 100) -> ()  [unwired: 1 out]
          }
          frame #2 {
            n523 = local read "Offset 2 Start (MHz)"() -> (w869:dbl)
            n524 = property on="Saved AOD Raster Scan Parameter Sets" class="Arr (strict)"("Index Values"=u32[] [2]) -> ()  [unwired: 2 in, 2 out]
            n525 = property on="Trap Delta (MHz)" class="DigNum (strict)"("Val(Sgnl)"=w869) -> ()  [unwired: 2 in, 2 out]
          }
          frame #3 {
            n526 = property on="Load parameters" class="Bool (strict)"("Val(Sgnl)"=TRUE ("Value (Signaling)")) -> ()  [unwired: 2 in, 2 out]
          }
          frame #4 {
            n527 = Wait (ms)(milliseconds to wait=u32 100) -> ()  [unwired: 1 out]
          }
          frame #5 {
            n528 = property on="Trap Raster Scan" class="Bool (strict)"("Val(Sgnl)"=TRUE ("Value (Signaling)")) -> ()  [unwired: 2 in, 2 out]
          }
          frame #6 {
            n529 = Wait (ms)(milliseconds to wait=u32 1000) -> ()  [unwired: 1 out]
          }
          frame #7 {
            n530 = while {
              stop <- w881 stop-if-true
              n531 = local read "Raster Scanning..."() -> (w883:bool)
              n532 = local read "Saving..."() -> (w882:bool)
              n533 = Not(x=w882) -> (.not. x?=w879:bool)
              n534 = Not(x=w883) -> (.not. x?=w880:bool)
              n535 = And(x=w880, y=w879) -> (x .and. y?=w881:bool)
            }
          }
          frame #8 {
            n536 = property on="Save ave N" class="DigNum (strict)"("Val(Sgnl)"=w884) -> ()  [unwired: 2 in, 2 out]
          }
        }
      }
      event "Step Size (nm)": Value Change {
        n537 = event-data() -> ()  [unwired: 1 in, 5 out]
        n538 = flat-sequence {
          frame #0 {
            n539 = property on="Saved AOD Raster Scan Parameter Sets" class="Arr (strict)"("Index Values"=u32[] [1]) -> ()  [unwired: 2 in, 2 out]
          }
          frame #1 {
            n540 = Multiply(x="N Steps", y="Step Size (nm)") -> (x*y=w886:dbl)
            n541 = property on="Scan Speed AOD (nm/s) 2" class="DigNum (strict)"("Value"="Step Size (nm)") -> ()  [unwired: 2 in, 2 out]
            n542 = property on="Step Size AOD (nm) 2" class="DigNum (strict)"("Value"="Step Size (nm)") -> ()  [unwired: 2 in, 2 out]
            n543 = property on="Scan Range AOD (nm) 2" class="DigNum (strict)"("Value"=w886) -> ()  [unwired: 2 in, 2 out]
          }
        }
      }
      event "Take Detection Laser\nImage": Value Change {
        n544 = event-data() -> ()  [unwired: 1 in, 5 out]
        n545 = flat-sequence {
          tunnel: [w914] -> w904
          tunnel: [w913] -> w897
          tunnel: [w912] -> w889
          tunnel: [w917] -> w905
          tunnel: w904 -> [w917]
          tunnel: [w916] -> w898
          tunnel: w897 -> [w916]
          tunnel: [w915] -> w890
          tunnel: w889 -> [w915]
          tunnel: [w921] -> w906
          tunnel: w905 -> [w921]
          tunnel: [w920] -> w899
          tunnel: w898 -> [w920]
          tunnel: [w919] -> w891
          tunnel: w890 -> [w919]
          tunnel: [w927] -> w907
          tunnel: w906 -> [w927]
          tunnel: [w926] -> w900
          tunnel: w899 -> [w926]
          tunnel: [w925] -> w892
          tunnel: w891 -> [w925]
          tunnel: [w931] -> w908
          tunnel: w907 -> [w931]
          tunnel: [w930] -> w901
          tunnel: w900 -> [w930]
          tunnel: [w929] -> w893
          tunnel: w892 -> [w929]
          tunnel: [w935] -> w909
          tunnel: w908 -> [w935]
          tunnel: [w934] -> w902
          tunnel: w901 -> [w934]
          tunnel: [w933] -> w894
          tunnel: w893 -> [w933]
          tunnel: [w939] -> w910
          tunnel: w909 -> [w939]
          tunnel: [w938] -> w903
          tunnel: w902 -> [w938]
          tunnel: [w937] -> w895
          tunnel: w894 -> [w937]
          tunnel: w910 -> [w945]
          tunnel: w903 -> [w944]
          tunnel: [w942] -> w896
          tunnel: w895 -> [w942]
          tunnel: w896 -> [w946]
          frame #0 {
            n546 = local read "Green Laser ON/Interlacing"() -> (w914:bool)
            n547 = local read "Green laser mode"() -> (w913:enum32{"Laser ON", "Laser OFF", "Interlace"})
            n548 = local read "Green FB On/Off"() -> (w912:bool)
          }
          frame #1 {
            n549 = property on="Green FB On/Off" class="Bool (strict)"("Val(Sgnl)"=FALSE ("Value (Signaling)")) -> ()  [unwired: 2 in, 2 out]
          }
          frame #2 {
            n550 = property on="Green Laser ON/Interlacing" class="Bool (strict)"("Val(Sgnl)"=TRUE ("Value (Signaling)")) -> ()  [unwired: 2 in, 2 out]
            n551 = property on="Flip Green Filter" class="Bool (strict)"("Val(Sgnl)"=TRUE ("Value (Signaling)")) -> ()  [unwired: 2 in, 2 out]
            n552 = property on="Green laser mode" class="RadioBtnsControl (strict)"("Val(Sgnl)"=enum32{"Laser ON", "Laser OFF", "Interlace"}."Laser ON" ("Value (Signaling)")) -> ()  [unwired: 2 in, 2 out]
          }
          frame #3 {
            n553 = Wait (ms)(milliseconds to wait=u32 500) -> ()  [unwired: 1 out]
          }
          frame #4 {
            n554 = property on="Confocal Image" class="Bool (strict)"("Val(Sgnl)"=TRUE ("Value (Signaling)")) -> ()  [unwired: 2 in, 2 out]
          }
          frame #5 {
            n555 = Wait (ms)(milliseconds to wait=u32 2000) -> ()  [unwired: 1 out]
          }
          frame #6 {
            n556 = while {
              stop <- w940 stop-if-true
              n557 = local read "Saving..."() -> (w941:bool)
              n558 = Not(x=w941) -> (.not. x?=w940:bool)
            }
          }
          frame #7 {
            n559 = property on="Flip Green Filter" class="Bool (strict)"("Val(Sgnl)"=TRUE ("Value (Signaling)")) -> ()  [unwired: 2 in, 2 out]
            n560 = property on="Green Laser ON/Interlacing" class="Bool (strict)"("Val(Sgnl)"=w945) -> ()  [unwired: 2 in, 2 out]
            n561 = property on="Green laser mode" class="RadioBtnsControl (strict)"("Val(Sgnl)"=w944) -> ()  [unwired: 2 in, 2 out]
          }
          frame #8 {
            n562 = property on="Green FB On/Off" class="Bool (strict)"("Val(Sgnl)"=w946) -> ()  [unwired: 2 in, 2 out]
          }
        }
      }
      event "Stop All": Value Change {
        n563 = event-data() -> ()  [unwired: 1 in, 5 out]
        n564 = local read "Stop All"() -> (w947:bool)
      }
    }
    n565 = node-c288() -> ()  [unwired: 1 in, 1 out]
  }
  n566 = node-c288(2 ("Processor")) -> (w20:T24)  [unwired: 3 in]
  n567 = timed-loop "Control parameters (event loop)" {
    tunnel: w2 -> [w951]
    shift-right: [w950] -> _
    shift-left: errorcluster {"status"=FALSE, "code"=0, "source"=""} ("error out") -> [w949]
    tunnel: [w948] -> w41
    timing: w20 -> [_]
    timing-out: [_] -> w19
    stop <- w948 stop-if-true
    n568 = node-c288() -> ()  [unwired: 1 in, 1 out]
    n569 = event shown="[6] \"BD 1 Frequency 1 (MHz)\", \"BD 1 Frequency 2 (MHz)\", \"BD 1 Frequency 3 (MHz)\", \"BD 2 Frequency 1 (MHz)\", \"BD 2 Frequency 2 (MHz)\", \"BD 2 Frequency 3 (MHz)\", \"Trap Delta (MHz)\": Value Change" {
      selector: _ -> [_ _ _ _ _ _ _ _ _ _ _ _ _ _ _ _ _ _ _ _ _ _ _ _ _ _ _ _ _ _ _ _ _ _ _ _ _ _ _ _ _ _ _ _ _ _ _ _ _ _ _ _ _ _ _ _]
      dyn-events: _ -> [_ _ _ _ _ _ _ _ _ _ _ _ _ _ _ _ _ _ _ _ _ _ _ _ _ _ _ _ _ _ _ _ _ _ _ _ _ _ _ _ _ _ _ _ _ _ _ _ _ _ _ _ _ _ _ _]
      timeout: _ -> [_ _ _ _ _ _ _ _ _ _ _ _ _ _ _ _ _ _ _ _ _ _ _ _ _ _ _ _ _ _ _ _ _ _ _ _ _ _ _ _ _ _ _ _ _ _ _ _ _ _ _ _ _ _ _ _]
      tunnel: w951 -> [w989 _ _ _ w1026 _ w1048 _ w1115 _ _ _ w1158 _ _ w1201 w1207 w1212 w1218 w1254 w1272 w1279 w1297 w1308 w1319 w1330 w1341 w1352 w1370 w1376 w1470 _ w1479 w1517 _ w1552 w1556 w1567 w1571 w1575 _ w1583 _ _ _ _ _ w1719 _ w1736 w1739 w1748 w1751 w1755 _ w1772]
      tunnel: [w988 _ _ _ w1016 _ w1047 _ w1078 _ w1123 _ w1137 _ _ w1200 w1203 w1209 w1215 w1253 w1270 w1278 w1291 w1302 w1313 w1324 w1335 w1346 w1368 w1375 w1468 _ w1477 w1515 _ w1550 w1554 w1557 w1569 w1573 _ w1581 _ _ _ _ _ w1717 _ _ _ _ _ _ _ _] -> w950
      tunnel: w949 -> [w987 _ _ _ w1025 _ w1046 _ w1110 _ w1123 _ w1157 _ _ w1199 w1202 w1208 w1214 w1252 w1271 w1277 w1296 w1307 w1318 w1329 w1340 w1351 w1369 w1374 w1469 _ w1478 w1516 _ w1551 w1555 w1566 w1570 w1574 _ w1582 _ _ _ _ _ w1718 _ w1735 w1738 w1747 w1750 w1754 _ w1771]
      tunnel: [_ _ _ _ _ _ _ _ _ _ w1122 _ _ _ _ _ _ _ _ _ _ _ _ _ _ _ _ _ _ _ _ _ _ _ _ _ _ _ _ _ _ _ _ _ _ _ _ _ _ _ _ _ _ _ _ _] -> w948
      tunnel: [_ _ _ _ _ _ _ "Round T1 X" _ _ _ _ _ _ _ _ _ _ _ _ _ _ _ _ _ _ _ _ _ _ _ _ _ _ _ _ _ _ _ _ _ _ _ _ _ _ _ _ _ _ _ _ _ _ _ _] -> _
      tunnel: [_ _ _ "Adjust Scale\nto Mean" _ _ _ _ _ _ _ _ _ _ _ _ _ _ _ _ _ _ _ _ _ _ _ _ _ _ _ _ _ _ _ _ _ _ _ _ _ _ _ _ _ _ _ _ _ _ _ _ _ "Set SP to Reading" _ _] -> _
      tunnel: [_ _ _ _ _ _ _ _ _ "Round T2 X" _ "Delayed Interlace Start" _ _ _ _ _ _ _ _ _ _ _ _ _ _ _ _ _ _ _ _ _ _ _ _ _ _ _ _ _ _ _ _ _ _ _ _ _ _ _ _ _ _ _ _] -> _
      event "AI Count (ticks)", "Sets to FIFO (Traps)", "Save ave N", "FPGA Ave.", "# Samples/channel", "N sets to save": Value Change {
        # "So that if 'Save ave N' is updated, the AOD scanning code updates too."
        n570 = event-data() -> ()  [unwired: 6 out]
        n571 = local read "AI Count (ticks)"() -> (w969:u32)
        n572 = Boolean To (0,1)(Boolean="Sets to FIFO (Traps)") -> (0, 1=w979:cluster{"Set 1":i16, "Set 2":i16, "Set 3":i16})
        n573 = xnode "Read/Write Control"("FPGA VI Reference In"=w989, "error in"=w987, "ai count"=w969, "AI1 Sets to FIFO"="Sets to FIFO (Traps)", "N of AI1 Int Acq Sets"="N Acq Sets (Traps + Fl.)") -> ("error out"=w988:errorcluster)  [unwired: 1 out]
        n574 = Cluster To Array(cluster=w979) -> (array=w978:i16[])
        n575 = To Unsigned Long Integer(number=w978) -> (unsigned 32bit integer=w958:u32[])
        n576 = local read "Scan steps (AOD)"() -> (w980:u64)
        n577 = Multiply(x=w969, y="N Acq Sets (Traps + Fl.)") -> (x*y=w967:u32)
        n578 = Divide(x=40000000.0, y=w969) -> (x/y=w961:dbl)
        "AI rate (Hz)" <- w961
        "Ave. Rate (Hz)" <- w961
        n579 = Add Array Elements(numeric array=w958) -> (sum=w970:u32)
        "Trap Sets" <- w970
        n580 = Reciprocal(x=w961) -> (1/x=→"Ave. Period (s)":dbl)
        n581 = property on="Scan steps (AOD)" class="DigNum (strict)"("Val(Sgnl)"=w980) -> ()  [unwired: 2 in, 2 out]
        n582 = Divide(x=w961, y="N Acq Sets (Traps + Fl.)") -> (x/y=w984:dbl)
        "Data Rate (Hz)" <- w984
        n583 = Reciprocal(x=w984) -> (1/x=→"Data Period (s)":dbl)
        n584 = local read "Save ave N"() -> (w983:dbl)
        n585 = Divide(x=w984, y=w983) -> (x/y=w982:dbl)
        "Save Data Rate (Hz)" <- w982
        n586 = Reciprocal(x=w982) -> (1/x=→"Save Data Period (s)":dbl)
        n587 = Multiply(x=w967, y="# Samples/trap") -> (x*y=w965:u32)
        "Counts/DMA" <- w965
        n588 = property on="Trap Disp. Downsample" class="DigNum (strict)"("Maximum"="# Samples/trap") -> ()  [unwired: 2 in, 2 out]
        n589 = Multiply(x=w970, y="# Samples/trap") -> (x*y=w959:u32)
        "# Samples/channel" <- w959
        n590 = Multiply(x=w959, y=u32 8) -> (x*y=→"Trap AI Elements/DMA read":u32)
        n591 = local read "APD Int. Count"() -> (w966:u32)
        n592 = Multiply(x=w959, y=u32 3) -> (x*y=→"Trap Pos Elements/DMA read":u32)
        n593 = Divide(x=w965, y=w966) -> (x/y=w956:dbl)
        "APD Samples/FIFO Acq." <- w956
        n594 = Divide(x=w965, y=40000000.0) -> (x/y=w963:dbl)
        "DMA Update Period (s)" <- w963
        n595 = Multiply(x=2.0, y=w956) -> (x*y=→"APD Elements/DMA read":dbl)
        n596 = property on="APD Disp. Downsample" class="DigNum (strict)"("Maximum"=w956) -> ()  [unwired: 2 in, 2 out]
        n597 = local read "N sets to save"() -> (w976:u32)
        n598 = Multiply(x=w963, y=w976) -> (x*y=→"Total Time (s)":dbl)
        "FPGA Averaging" <- FALSE ("FPGA Averaging")
      }
      event "Rescale on Mean": Value Change {
        n599 = event-data() -> ()  [unwired: 7 out]
        n600 = And(x=FALSE, y="Rescale on Mean") -> (x .and. y?=w991:bool)
        n601 = local write "Rescale on Mean"(w991) -> ()
        n602 = local read "Bead Mean (nm)"() -> (w996:dbl)
        n603 = Add(x="Amplitude (nm)", y=w996) -> (x+y=w994:dbl)
        n604 = Subtract(x=w996, y="Amplitude (nm)") -> (x-y=w993:dbl)
        n605 = property on="Bead Separation" class="WFChart (strict)"("YScale.Minimum"=w993) -> ()  [unwired: 2 in, 2 out]
        n606 = property on="Bead Separation" class="WFChart (strict)"("YScale.Maximum"=w994) -> ()  [unwired: 2 in, 2 out]
      }
      event "Detector Type": Value Change {
        n607 = event-data() -> ()  [unwired: 7 out]
        n608 = local read "AI labels"() -> (w997:string[])
        n609 = property on="High Res. Display" class="Ring (strict)"("Strings []"=w997) -> ()  [unwired: 2 in, 2 out]
        n610 = Build Array (concatenate)(w997, "none") -> (w998:string[])
        n611 = property on="FFT 1 Choice 1" class="Ring (strict)"("Strings []"=w998) -> ()  [unwired: 2 in, 2 out]
        n612 = property on="FFT 1 Choice 2" class="Ring (strict)"("Strings []"=w998) -> ()  [unwired: 2 in, 2 out]
        n613 = property on="FFT 2 Choice 1" class="Ring (strict)"("Strings []"=w998) -> ()  [unwired: 2 in, 2 out]
        n614 = property on="FFT 2 Choice 2" class="Ring (strict)"("Strings []"=w998) -> ()  [unwired: 2 in, 2 out]
        n615 = Bundle("APD 1", "APD 2") -> (w1001:cluster{string, string})  [unwired: 1 out]
        n616 = Cluster To Array(cluster=w1001) -> (array=w999:string[])
        n617 = Build Array (concatenate)(w999, w998) -> (w1003:string[])
        n618 = Array Size(array=w1003) -> (size(s)=w1004:i32)
        n619 = property on="Signals to Plot" class="LstBox (strict)"("Item Names"=w1003) -> ()  [unwired: 2 in, 2 out]
        n620 = property on="Signals to Plot" class="LstBox (strict)"("Number of Rows"=w1004) -> ()  [unwired: 2 in, 2 out]
        n621 = property on="All Signals" class="WFChart (strict)"("LegNumRows"=w1004) -> ()  [unwired: 2 in, 2 out]
      }
      event "Adjust Scale\nto Mean": Value Change {
        n622 = event-data() -> ()  [unwired: 7 out]
        n623 = local read "APD 1 Rate (Hz)"() -> (w1013:dbl)
        n624 = Multiply(x=1000.0, y="Above (kHz)") -> (x*y=w1011:dbl)
        n625 = Multiply(x=1000.0, y="Below (kHz)") -> (x*y=w1009:dbl)
        n626 = Add(x=w1011, y=w1013) -> (x+y=w1006:dbl)
        n627 = Subtract(x=w1013, y=w1009) -> (x-y=w1007:dbl)
        n628 = property on="APD Chart" class="WFChart (strict)"("YScale.Minimum"=w1007) -> ()  [unwired: 2 in, 2 out]
        n629 = property on="APD Chart" class="WFChart (strict)"("YScale.Maximum"=w1006) -> ()  [unwired: 2 in, 2 out]
      }
      event "Phase adj. (AI1)", "+ phase (AI1)", "- phase (AI1)": Value Change {
        n630 = event-data() -> ()  [unwired: 7 out]
        n631 = Negate(x="Phase adj. (AI1)") -> (-x=w1023:i16)
        n632 = Select(t=w1023, s="- phase (AI1)", f="Phase adj. (AI1)") -> (s? t:f=w1022:i16)
        n633 = xnode "Read/Write Control"("FPGA VI Reference In"=w1026, "error in"=w1025, "Phase count adjustment"=w1022) -> ("FPGA VI Reference Out"=w1021:T19, "error out"=w1020:errorcluster)
        n634 = Or(x="- phase (AI1)", y="+ phase (AI1)") -> (x .or. y?=w1017:bool)
        n635 = xnode "Read/Write Control"("FPGA VI Reference In"=w1021, "error in"=w1020, "+ phase"=w1017) -> ("error out"=w1016:errorcluster)  [unwired: 1 out]
      }
      event "Signals to Plot": Double Click {
        w1029 = u32 9868950 ("Color Box")
        n636 = event-data() -> ("Row"=w1031:i32)  [unwired: 9 out]
